vi "Append Text Table to Report.vi"(0 "report in":refnum<class "NI_Word.lvclass">, 1 "column width (1)":dbl=1.0 format="%.2f", 2 "measurement system":u16(ring)=2 caption="measurement system for column width (Default)" items=["US", "Metric", "Default"], 3 "MS Office parameters":T2, 5 "column headers":string[](array[string]), 7 "row headers":string[](array[string]), 9 "text data":string[][](array[string]), 11 "error in (no error)":errorcluster, 13 "separate page?":bool, 14 "show grid lines":bool=TRUE) -> (4 "report out":refnum<class "NI_Word.lvclass">, 8 "range (wd) - start (xl)":T1, 10 "end (xl)":cluster{"row (xl) ":i32, "col (xl) ":i32}, 15 "error out":errorcluster)   [LabVIEW 2015, in "NI_Word.lvclass"]
doc: "Appends a 2D array to a report as a table with the given column width. You can use this polymorphic VI to append an array of strings or numbers. The data type you wire to the <B>text data</B> input determines the polymorphic instance to use."
uses:
  <vilib>/Utility/NIReport.llb/Word/NI_Word.lvclass
  <vilib>/Utility/NIReport.llb/Word/NI_Word.lvclass/NI_Word.ctl
  <vilib>/addons/_office/NI_ReportGenerationToolkit.lvlib
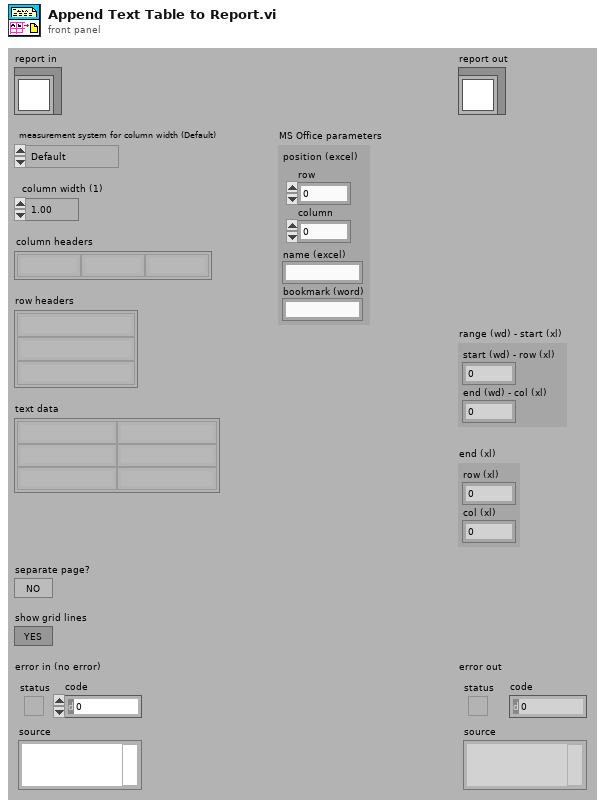
[diagram p1: front panel]
types:
  T1 = cluster{"start (wd) - row (xl) ":i32, "end (wd) - col (xl) ":i32}
  T2 = cluster{"position (excel)":cluster{"row":i32, "column":i32}, "name (excel)":string, "bookmark (word)":string}
  T3 = typedef "NI_ReportGenerationCore.lvlib/Report Data Members.ctl" = cluster{"font":T4, "from template?":bool}
  T4 = typedef "NI_ReportGenerationCore.lvlib/font.ctl" = cluster{"font name":string, "font size":dbl, "bold":u16, "italic":u16, "underline":u16, "strike through":u16, "font color":u32}
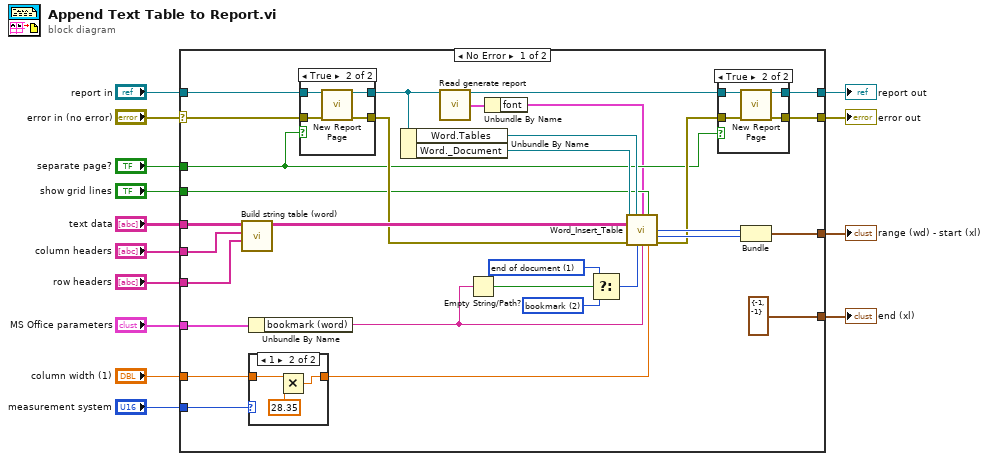
[diagram p0: block diagram]
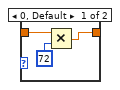
[diagram p2: hidden frame]
diagram:
  n1 = case shown="No Error" "error in (no error)" {
    selector: "error in (no error)" -> [w30 w65]
    tunnel: [w29 w65] -> w13
    tunnel: [w32 w64] -> w11
    tunnel: "report in" -> [w34 w64]
    tunnel: "MS Office parameters" -> [w28 _]
    tunnel: "show grid lines" -> [w27 _]
    tunnel: "separate page?" -> [w26 _]
    tunnel: "text data" -> [w25 _]
    tunnel: "column headers" -> [w24 _]
    tunnel: "row headers" -> [w23 _]
    tunnel: "measurement system" -> [w22 _]
    tunnel: [w21 _] -> w3
    tunnel: [cluster{"row (xl)":i32, "col (xl)":i32} {"row (xl)"=-1, "col (xl)"=-1} ("end (xl)") _] -> w2
    tunnel: "column width (1)" -> [w19 _]
    frame No Error {
      w35 = u16 2 items=["begining of document", "end of document", "bookmark", "custom"] ("Insertion point")
      w36 = u16 1 items=["begining of document", "end of document", "bookmark", "custom"] ("Insertion point")
      n2 = call <vilib>:"Build string table (word).vi"("row headers"=w23, "column headers"=w24, "text data"=w25) -> ("output table"=w41:string[][])  [unwired: 1 in, 7 out]
      n3 = Unbundle By Name(w28) -> ("bookmark (word)"=w39:string)
      n4 = case shown="1" w22 {
        tunnel: w19 -> [w48 w50]
        tunnel: [w47 w49] -> w38
        frame 0, Default {
          n5 = Multiply(x=w48, y=72) -> (x*y=w47:dbl)
        }
        frame 1 {
          n6 = Multiply(x=w50, y=28.35) -> (x*y=w49:dbl)
        }
      }
      n7 = case shown="True" w26 {
        tunnel: w34 -> [w59 w63]
        tunnel: w30 -> [w58 w62]
        tunnel: [w59 w60] -> w18
        tunnel: [w58 w61] -> w33
        frame False {
        }
        frame True {
          n8 = call-dynamic "New Report Page.vi"("report in"=w63, "error in (no error)"=w62) -> ("report out"=w60:refnum<class "NI_Word.lvclass">, "error out"=w61:errorcluster)  [unwired: 12 in]
        }
      }
      n9 = Unbundle By Name(w18) -> ("Word.Tables"=w42:refnum<k7>, "Word._Document"=w40:refnum<k7>)
      n10 = call-dynamic "Read generate report.vi"("report in"=w18) -> ("report out"=w17:refnum<class "NI_Word.lvclass">, "generate report"=w16:T3)  [unwired: 12 in, 1 out]
      n11 = Empty String/Path?(string/path=w39) -> (empty?=w37:bool)
      n12 = Unbundle By Name(w16) -> ("font"=w15:T4)
      n13 = Select(t=w36, s=w37, f=w35) -> (s? t:f=w43:u16)
      n14 = call <vilib>:"Word_Insert_Table.vi"("Document"=w40, "Tables"=w42, "font"=w15, "show grid lines"=w27, "Table data"=w41, "error in (no error)"=w33, "Insertion point"=w43, "Bookmark name"=w39, "column width (1)"=w38) -> ("Start out"=w44:i32, "End out"=w45:i32, "error out"=w31:errorcluster)  [unwired: 2 in, 2 out]
      n15 = case shown="True" w26 {
        tunnel: [w53 w57] -> w32
        tunnel: [w52 w56] -> w29
        tunnel: w31 -> [w52 w55]
        tunnel: w17 -> [w53 w54]
        frame False {
        }
        frame True {
          n16 = call-dynamic "New Report Page.vi"("report in"=w54, "error in (no error)"=w55) -> ("report out"=w57:refnum<class "NI_Word.lvclass">, "error out"=w56:errorcluster)  [unwired: 12 in]
        }
      }
      n17 = Bundle("Start out"=w44, "End out"=w45) -> (w21:cluster{"Start out":i32, "End out":i32})  [unwired: 1 out]
    }
    frame Error {
    }
  }
  "error out" <- w13
  "report out" <- w11
  "end (xl)" <- w2
  "range (wd) - start (xl)" <- w3
